vi "Write Key.vi"(8 "error in (no error)":errorcluster, 9 "Value":string, 10 "Key":string, 11 "E2E editor node in":refnum<data-value>) -> (0 "error out":errorcluster, 3 "E2E editor node out":refnum<data-value>)   [LabVIEW 2015, in "E2E Tag Exchange editor node.lvclass"]
uses:
  E2E Tag Exchange editor node.lvclass
  module/configuration/E2E Tag Exchange configuration.lvclass
  <vilib>/NI/Configuration Framework/serializable configuration/NISE_CEF_serializable configuration.lvclass
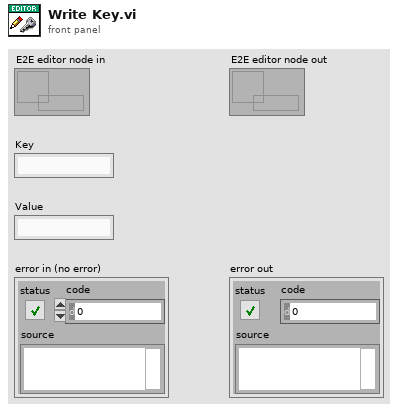
[diagram p1: front panel]
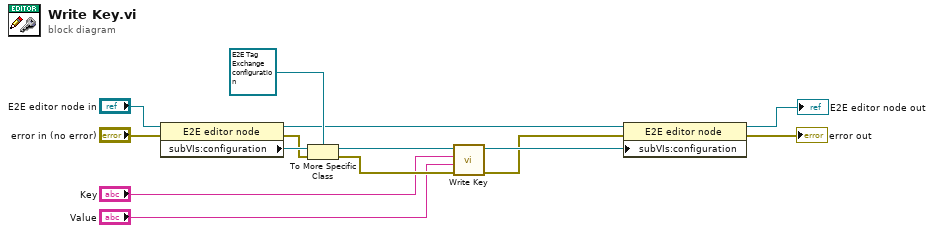
[diagram p0: block diagram]
diagram:
  n1 = property class="E2E editor node"(reference="E2E editor node in", error in="error in (no error)") -> (reference out=w9:refnum<data-value>, error out=w12:errorcluster, "subVIs:configuration"=w13:refnum<class "NISE_CEF_serializable configuration.lvclass">)
  n2 = To More Specific Class(target class=refnum<class "E2E Tag Exchange configuration.lvclass"> refnum ("E2E configuration"), reference=w13, error in=w12) -> (specific class reference=w5:refnum<class "E2E Tag Exchange configuration.lvclass">, error out=w6:errorcluster)
  n3 = call "Write Key.vi"("error in"=w6, "Value"="Value", "Key"="Key", "E2E configuration in"=w5) -> ("error out"=w3:errorcluster, "E2E configuration out"=w4:refnum<class "E2E Tag Exchange configuration.lvclass">)  [unwired: 6 in]
  n4 = property class="E2E editor node"(reference=w9, error in=w3, "subVIs:configuration"=w4) -> (reference out=→"E2E editor node out":refnum<data-value>, error out=→"error out":errorcluster)
